vi "Display.vi"(8 "error in":errorcluster, 11 "Plain - One Button in":refnum<class "Plain - One Button.lvclass">) -> (0 "error out":errorcluster, 3 "Plain - One Button out":refnum<class "Plain - One Button.lvclass">)   [LabVIEW 2021, in "Pop-Up.lvlib" / "Plain - One Button.lvclass"]
doc: "This is the override method required for each child of the pop up class. It is the pop up that will display to the user.\n\nTo extend this function, create a child class of the pop up class. Then create an override method for this VI. <b>Display.vi</b> is a protected function, therefore it cannot be called in a main application. This VI must be called by a caller function. See one of the standard pop-ups for a setup example.\n\n<b>Code Developed By:</b> +\nDaniel Coons +\nhttps://github.com/danielcoons/tsc-pop-up"
uses:
  Plain - One Button.lvclass
  C:/Development/Open Source/tsc-pop-up/Popup/Popup.lvclass
  C:/Development/Open Source/tsc-pop-up/Plain/Plain Parent.lvclass
  Popup/Popup.lvclass/Popup.ctl
  Plain Parent.lvclass/Plain Parent.ctl
  Popup/Data Member Access/Read Theme.vi
  Get Transparent buttons.vi
  Get Dialog Title.vi
  Get Action 1 Text.vi
  Theme/Theme.lvclass
  Plain - One Button.lvclass/Plain - One Button.ctl
  Popup/Popup.lvclass
  user32.dll
panel:
  out "dialog title":string
  out "message":string
  in  "action 1":bool
  # "This VI displays the popup"
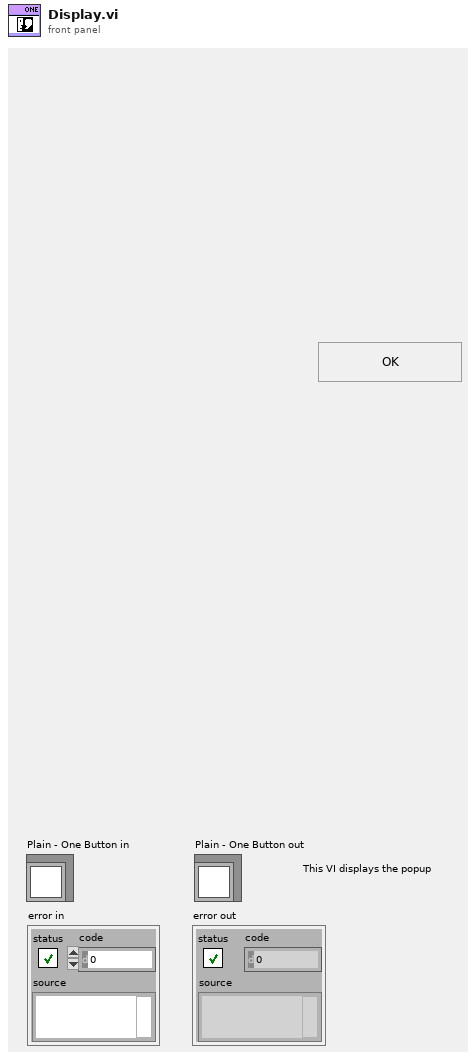
[diagram p1: front panel]
types:
  T1 = typedef "LVRectTypeDef.ctl" = cluster{"Left":i16, "Top":i16, "Right":i16, "Bottom":i16}
  T2 = typedef "LVPointTypeDef.ctl" = cluster{"Horizontal":i16, "Vertical":i16}
  T3 = typedef "LVPoint32TypeDef.ctl" = cluster{"Horizontal":i32, "Vertical":i32}
  T4 = typedef "LVPositionTypeDef.ctl" = cluster{"Left":i32, "Top":i32}
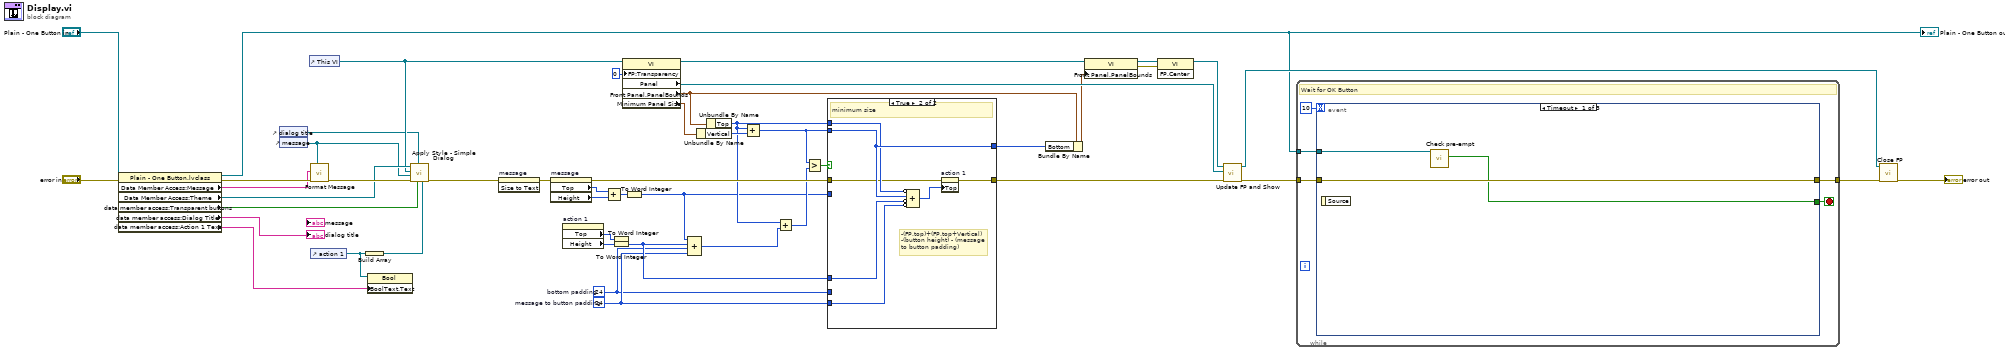
[diagram p0: block diagram]
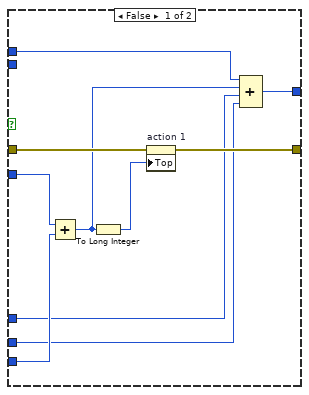
[diagram p2: hidden frame]
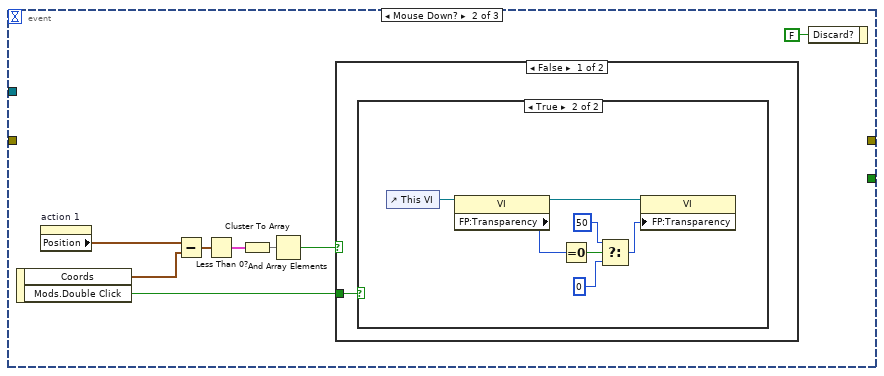
[diagram p3: hidden frame]
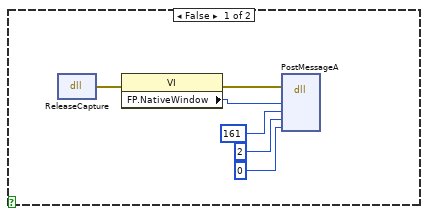
[diagram p4: hidden frame]
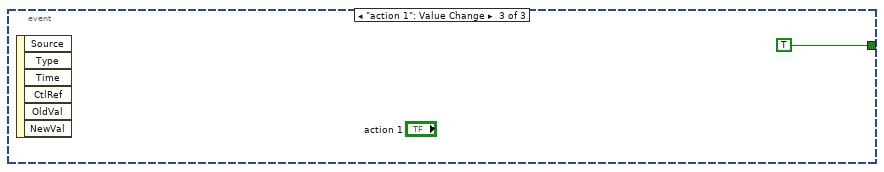
[diagram p6: hidden frame]
diagram:
  w20 = i16 24  # message to button padding
  w18 = i16 24  # bottom padding
  n1 = property class="Plain - One Button.lvclass"(reference="Plain - One Button in", error in="error in") -> (reference out=w2:refnum<class "Plain - One Button.lvclass">, error out=w43:errorcluster, "Data Member Access:Message"=w39:string, "Data Member Access:Theme"=w12:refnum<class "Theme.lvclass">, "data member access:Transparent buttons"=w1:bool, "data member access:Dialog Title"=→"dialog title":string, "data member access:Action 1 Text"=w7:string)
  "Plain - One Button out" <- w2
  n2 = control-ref of="dialog title"() -> (w6:refnum<vi>)
  n3 = control-ref of="message"() -> (w5:refnum<vi>)
  n4 = control-ref of="This VI"() -> (w11:refnum<vi>)
  n5 = call "Format Message.vi"("formatted string"=w5, "error in"=w43, "String Input"=w39) -> ("error out"=w14:errorcluster)  [unwired: 7 in, 1 out]
  n6 = control-ref of="action 1"() -> (w8:refnum<vi>)
  n7 = Build Array(w8) -> (w10:refnum<vi>[])
  n8 = property class="Bool"(reference=w8, "BoolText.Text"=w7) -> ()  [unwired: 1 in, 2 out]
  n9 = call "Apply Style - Simple Dialog.vi"("button refs"=w10, "keep transparent buttons?"=w1, "title ref"=w6, "error in"=w14, "message ref"=w5, "pop up ref"=w11, "Theme in"=w12) -> ("error out"=w13:errorcluster)  [unwired: 3 in, 1 out]
  n10 = invoke on="message" class="Str" method="Size to Text"(error in=w13) -> (error out=w42:errorcluster)  [unwired: 2 in, 2 out]
  n11 = property on="message" class="Str"(error in=w42) -> (error out=w23:errorcluster, "Top"=w34:i32, "Height"=w33:u32)  [unwired: 1 in, 1 out]
  n12 = property on="action 1" class="Bool"() -> ("Top"=w36:i32, "Height"=w35:u32)  [unwired: 2 in, 2 out]
  n13 = Add(x=w34, y=w33) -> (x+y=w32:u32)
  n14 = To Word Integer(number=w36) -> ()  [unwired: 1 out]
  n15 = To Word Integer(number=w35) -> (16bit integer=w21:i16)
  n16 = property class="VI"(reference=w11, "FP:Transparency"=u8 0 ("Front Panel Window:Transparency")) -> (reference out=w38:refnum<vi>, "Panel"=w37:refnum<vi>, "Front Panel.PanelBounds"=w28:T1, "Minimum Panel Size"=w31:T2)  [unwired: 1 in, 1 out]
  n17 = To Word Integer(number=w32) -> (16bit integer=w3:i16)
  n18 = Compound Arithmetic op=ADD(w3, w21, w18, w20) -> (w4:i16)
  n19 = Unbundle By Name(w31) -> ("Vertical"=w30:i16)
  n20 = Unbundle By Name(w28) -> ("Top"=w15:i16)
  n21 = Add(x=w15, y=w30) -> (x+y=w16:i16)
  n22 = Add(x=w15, y=w4) -> (x+y=w17:i16)
  n23 = Greater?(x=w16, y=w17) -> (0:w24:bool)
  n24 = case shown="True" w24 {
    tunnel: [w57 w64] -> w19
    tunnel: w16 -> [_ w64]
    tunnel: w3 -> [w58 _]
    tunnel: w15 -> [w49 w63]
    tunnel: w23 -> [w56 w62]
    tunnel: [w53 w61] -> w22
    tunnel: w21 -> [w51 w60]
    tunnel: w20 -> [w55 w59]
    tunnel: w18 -> [w52 _]
    frame False {
      n25 = Add(x=w58, y=w55) -> (x+y=w50:i16)
      n26 = To Long Integer(number=w50) -> (32bit integer=w54:i32)
      n27 = property on="action 1" class="Bool"(error in=w56, "Top"=w54) -> (error out=w53:errorcluster)  [unwired: 1 in, 1 out]
      n28 = Compound Arithmetic op=ADD(w49, w50, w51, w52) -> (w57:i16)
    }
    frame True {
      # "-(FP.top)+(FP.top+Vertical)\n-(button height) - (message\nto button padding)"
      # "minimum size"
      n29 = Compound Arithmetic op=ADD(invert w63, w64, invert w60, invert w59) -> (w65:i16)
      n30 = property on="action 1" class="Bool"(error in=w62, "Top"=w65) -> (error out=w61:errorcluster)  [unwired: 1 in, 1 out]
    }
  }
  n31 = Bundle By Name(cluster=w28, "Bottom"=w19) -> (w25:T1)
  n32 = property class="VI"(reference=w38, "Front Panel.PanelBounds"=w25) -> (reference out=w29:refnum<vi>, error out=w26:errorcluster)  [unwired: 1 in]
  n33 = invoke class="VI" method="FP.Center"(reference=w29, error in=w26) -> (reference out=w27:refnum<vi>)  [unwired: 1 in, 2 out]
  n34 = call "Update FP and Show.vi"("error in (no error)"=w22, "Panel Ref"=w37, "VI in"=w27) -> ("error out"=w47:errorcluster, "VI out"=w46:refnum<vi>)  [unwired: 7 in]
  n35 = while {
    tunnel: [w68] -> w48
    tunnel: w47 -> [w69]
    tunnel: w2 -> [w66]
    stop <- w70 stop-if-true
    # "Wait for OK Button"
    n36 = event shown="[0] Timeout" {
      selector: _ -> [_ _ _]
      dyn-events: _ -> [_ _ _]
      timeout: 10 -> [_ _ _]
      tunnel: [w71 _ TRUE ("Pre-empted?")] -> w70
      tunnel: w69 -> [w73 _ _]
      tunnel: [w73 _ _] -> w68
      tunnel: w66 -> [w72 _ _]
      event Timeout {
        n37 = event-data() -> ()  [unwired: 1 in, 1 out]
        n38 = call "Check pre-empt.vi"("_Popup in"=w72) -> ("Pre-empted?"=w71:bool)  [unwired: 8 in, 2 out]
      }
      event Mouse Down? {
        n39 = event-data() -> ("Coords"=w75:T3, "Mods.Double Click"=w77:bool)  [unwired: 1 in]
        n40 = property on="action 1" class="Bool"() -> ("Position"=w76:T4)  [unwired: 2 in, 2 out]
        n41 = Subtract(x=w76, y=w75) -> (x-y=w78:T4)
        n42 = Less Than 0?(x=w78) -> (x < 0?=w79:cluster{"Left":bool, "Top":bool})
        n43 = Cluster To Array(cluster=w79) -> (array=w80:bool[])
        n44 = And Array Elements(Boolean array=w80) -> (logical AND=w81:bool)
        n45 = case shown="False" w81 {
          tunnel: w77 -> [w82 _]
          frame False {
            n46 = case shown="True" w82 {
              frame False {
                n47 = dll-call lib="user32.dll" fn="ReleaseCapture"() -> (error out=w86:errorcluster)  [unwired: 4 in, 1 out]
                n48 = property class="VI"(error in=w86) -> (error out=w87:errorcluster, "FP.NativeWindow"=w88:u64)  [unwired: 1 in, 1 out]
                n49 = dll-call lib="user32.dll" fn="PostMessageA"(error in=w87, "hWnd"=w88, "Msg"=161, "wParam"=2, "lParam"=0) -> ()  [unwired: 7 in, 2 out]
              }
              frame True {
                n50 = control-ref of="This VI"() -> (w95:refnum<vi>)
                n51 = property class="VI"(reference=w95) -> (reference out=w93:refnum<vi>, "FP:Transparency"=w94:u8)  [unwired: 1 in, 1 out]
                n52 = Equal To 0?(x=w94) -> (x = 0?=w92:bool)
                n53 = Select(t=u8 50, s=w92, f=u8 0) -> (s? t:f=w91:u8)
                n54 = property class="VI"(reference=w93, "FP:Transparency"=w91) -> ()  [unwired: 1 in, 2 out]
              }
            }
          }
          frame True {
          }
        }
        n55 = event-data("Discard?"=FALSE) -> ()  [unwired: 1 in, 1 out]
      }
      event "action 1": Value Change {
        n56 = event-data() -> ()  [unwired: 1 in, 6 out]
      }
    }
  }
  n57 = call "Close FP.vi"("error in (no error)"=w48, "VI in"=w46) -> ("error out"=→"error out":errorcluster)  [unwired: 9 in]
